vi "GetExcelData.vi"(7 "Format":enum16{"string", "numeral"}(ring), 8 "error":errorcluster caption="错误输入（无错误）", 9 "SecondCell":string, 10 "FirstCell":string, 11 "Excel._Worksheet":refnum<k7>) -> (0 "error out":errorcluster caption="错误输出", 1 "Data(Numeral)":sgl[][](array[numeric]), 2 "Data(string)":string[][](array[string]), 3 "Excel._Worksheet":refnum<k7>)   [LabVIEW 2017]
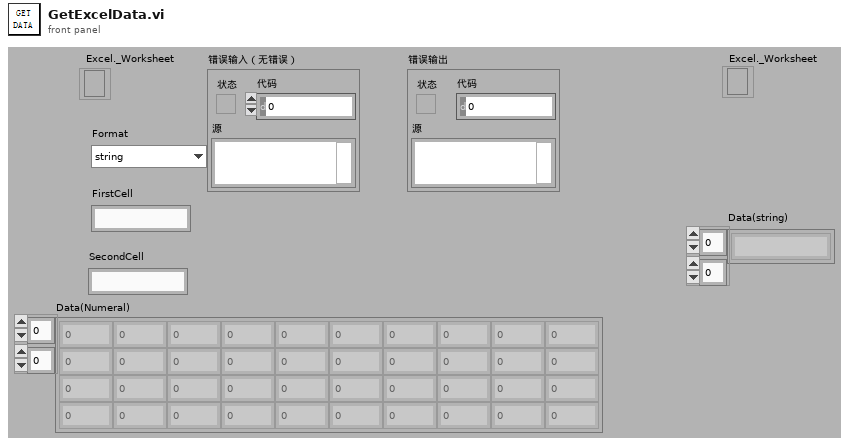
[diagram p1: front panel]
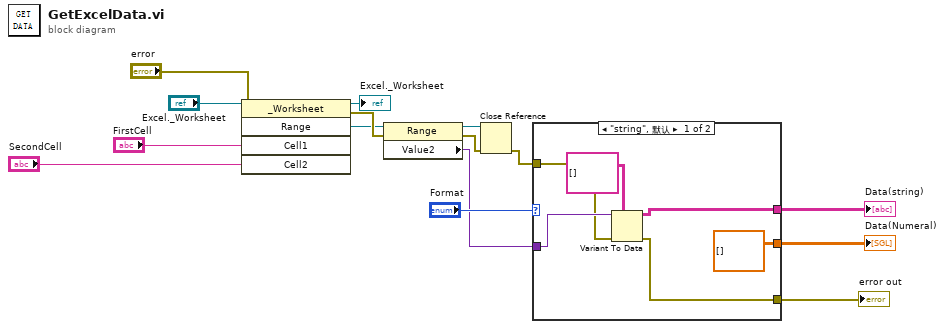
[diagram p0: block diagram]
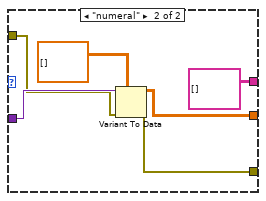
[diagram p2: hidden frame]
diagram:
  n1 = invoke class="_Worksheet" method="Range"(reference="Excel._Worksheet", error in="error", "Cell1"="FirstCell", "Cell2"="SecondCell") -> (reference out=→"Excel._Worksheet":refnum<k7>, error out=w15:errorcluster, "Range"=w4:refnum<k7>)  [unwired: 1 in, 2 out]
  n2 = property class="Range"(reference=w4, error in=w15) -> (reference out=w3:refnum<k7>, error out=w2:errorcluster, "Value2"=w13:variant)
  n3 = Close Reference(reference=w3, error in (no error)=w2) -> (error out=w1:errorcluster)
  n4 = case shown="\"string\", 默认" "Format" {
    tunnel: w13 -> [w21 w26]
    tunnel: [sgl[][] [] w25] -> w12
    tunnel: [w18 string[][] []] -> w11
    tunnel: [w16 w23] -> w10
    tunnel: w1 -> [w17 w22]
    frame "string", Default {
      n5 = Variant To Data(error in=w17, type=string[][] [], Variant=w21) -> (data=w18:string[][], error out=w16:errorcluster)
    }
    frame "numeral" {
      n6 = Variant To Data(error in=w22, type=sgl[][] [], Variant=w26) -> (data=w25:sgl[][], error out=w23:errorcluster)
    }
  }
  "error out" <- w10
  "Data(Numeral)" <- w12
  "Data(string)" <- w11
